vi "ReadNumeric.vi"(1 "reference":refnum<vi>) -> (0 "Numeric":T10)   [LabVIEW 2013]
uses:
  <vilib>/Utility/miscctls.llb/LVBoundsTypeDef.ctl
  <vilib>/Utility/miscctls.llb/LVRectTypeDef.ctl
  <vilib>/Utility/miscctls.llb/LVPositionTypeDef.ctl
  <vilib>/Utility/miscctls.llb/LVDataSocketStatusTypeDef.ctl
  <vilib>/Utility/miscctls.llb/LVKeyNavTypeDef.ctl
  <vilib>/Utility/miscctls.llb/LVMinMaxIncTypeDef.ctl
  <vilib>/Utility/miscctls.llb/LVKeyTypeDef.ctl
  <vilib>/numeric/LVNumericRepresentation.ctl
  <vilib>/Utility/miscctls.llb/LVOutOfRangeActionTypeDef.ctl
panel:
  out "error out":errorcluster
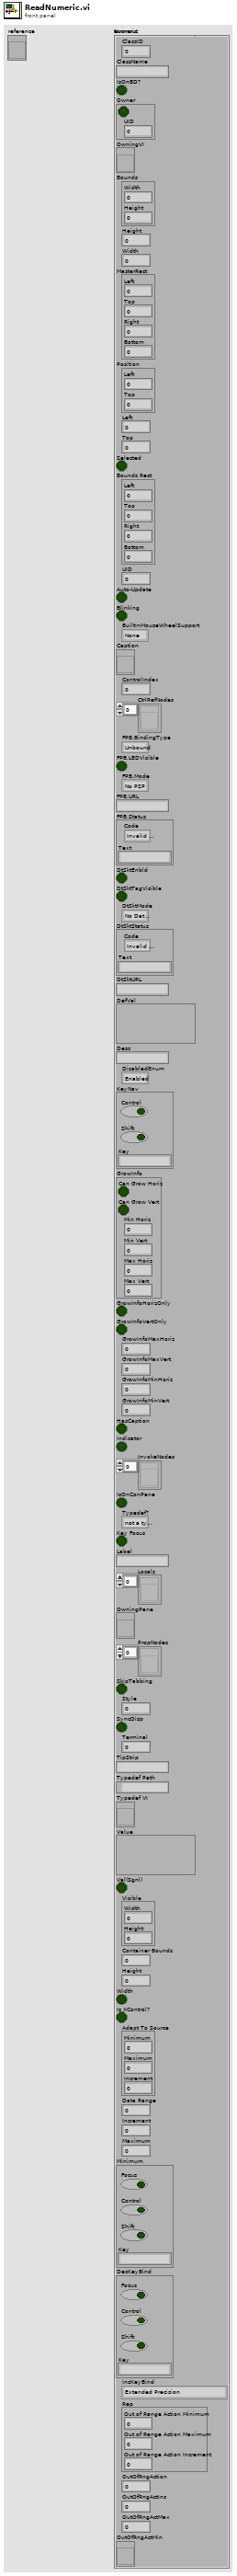
[diagram p1: front panel]
types:
  T1 = typedef "LVBoundsTypeDef.ctl" = cluster{"Width":u32, "Height":u32}
  T2 = typedef "LVRectTypeDef.ctl" = cluster{"Left":i16, "Top":i16, "Right":i16, "Bottom":i16}
  T3 = typedef "LVPositionTypeDef.ctl" = cluster{"Left":i32, "Top":i32}
  T4 = typedef "LVDataSocketStatusTypeDef.ctl" = cluster{"Code":enum32{"Invalid Status", "Unconnected", "Active", "Idle", "Error", "Connecting"}, "Text":string}
  T5 = typedef "LVKeyNavTypeDef.ctl" = cluster{"Control":bool, "Shift":bool, "Key":string}
  T6 = typedef "LVMinMaxIncTypeDef.ctl" = cluster{"Minimum":dbl, "Maximum":dbl, "Increment":dbl}
  T7 = typedef "LVKeyTypeDef.ctl" = cluster{"Focus":bool, "Control":bool, "Shift":bool, "Key":string}
  T8 = typedef "LVNumericRepresentation.ctl" = enum32{"Extended Precision", "Double Precision", "Single Precision", "Long", "Word", "Byte", "Unsigned Long", "Unsigned Word", "Unsigned Byte", "Complex Extended", "Complex Double", "Complex Single", "Quad", "Unsigned Quad", "Fixed-Point"}
  T9 = typedef "LVOutOfRangeActionTypeDef.ctl" = cluster{"Out of Range Action Minimum":u8, "Out of Range Action Maximum":u8, "Out of Range Action Increment":u8}
  T10 = cluster{"ClassID":u32, "ClassName":string, "IsOnBD?":bool, "Owner":cluster{bool, "UID":i32}, "OwningVI":refnum<vi>, "Bounds":T1, "Height":u32, "Width":u32, "MasterRect":T2, "Position":T3, "Left":i32, "Top":i32, "Selected":bool, "Bounds Rect":T2, "UID":i32, "Auto-Update":bool, "Blinking":bool, "BuiltInMouseWheelSupport":enum16{"None", "On Hover", "On Key Focus", "On Hover or Key Focus"}, "Caption":refnum<vi>, "ControlIndex":i32, "CtrlRefNodes":refnum<vi>[], "FPB.BindingType":enum32{"Unbound", "Bound To PSP URL", "Bound To Variable Shortcut"}, "FPB.LEDVisible":bool, "FPB.Mode":enum32{"No PSP", "Read", "Write", "Write & Read"}, "FPB.URL":string, "FPB.Status":T4, "DtSktEnbld":bool, "DtSktTagVisible":bool, "DtSktMode":enum32{"No DataSocket", "Publish", "Subscribe", "Publish & Subscribe"}, "DtSktStatus":T4, "DtSktURL":string, "DefVal":variant, "Desc":string, "DisabledEnum":enum8{"Enabled", "Disabled", "Disabled and Grayed Out"}, "KeyNav":T5, "GrowInfo":cluster{"Can Grow Horiz":bool, "Can Grow Vert":bool, "Min Horiz":i16, "Min Vert":i16, "Max Horiz":i16, "Max Vert":i16}, "GrowInfoHorizOnly":bool, "GrowInfoVertOnly":bool, "GrowInfoMaxHoriz":i16, "GrowInfoMaxVert":i16, "GrowInfoMinHoriz":i16, "GrowInfoMinVert":i16, "HasCaption":bool, "Indicator":bool, "InvokeNodes":refnum<vi>[], "IsOnConPane":bool, "Typedef?":enum32{"not a typedef", "typedef", "strict typedef", "class private data"}, "Key Focus":bool, "Label":string, "Locals":refnum<vi>[], "OwningPane":refnum<vi>, "PropNodes":refnum<vi>[], "SkipTabbing":bool, "Style":u32, "SyncDisp":bool, "Terminal":i32, "TipStrip":string, "Typedef Path":path, "Typedef VI":refnum<vi>, "Value":variant, "Val(Sgnl)":bool, "Visible":T1, "Container Bounds":u32, "Height":u32, "Width":bool, "Is XControl?":bool, "Adapt To Source":T6, "Data Range":dbl, "Increment":dbl, "Maximum":dbl, "Minimum":T7, "DecKeyBind":T7, "IncKeyBind":T8, "Rep":T9, "OutOfRngAction":u8, "OutOfRngActInc":u8, "OutOfRngActMax":u8, "OutOfRngActMin":refnum<vi>}
  T11 = enum16{"None", "On Hover", "On Key Focus", "On Hover or Key Focus"}
  T12 = enum32{"Unbound", "Bound To PSP URL", "Bound To Variable Shortcut"}
  T13 = enum32{"No PSP", "Read", "Write", "Write & Read"}
  T14 = enum32{"No DataSocket", "Publish", "Subscribe", "Publish & Subscribe"}
  T15 = enum8{"Enabled", "Disabled", "Disabled and Grayed Out"}
  T16 = cluster{"Can Grow Horiz":bool, "Can Grow Vert":bool, "Min Horiz":i16, "Min Vert":i16, "Max Horiz":i16, "Max Vert":i16}
  T17 = enum32{"not a typedef", "typedef", "strict typedef", "class private data"}
  T18 = cluster{"ClassID":u32, "ClassName":string, "IsOnBD?":bool, "Cluster":cluster{bool, "UID":i32}, "OwningVI":refnum<vi>, "Bounds":T1, "Height":u32, "Width":u32, "MasterRect":T2, "Position":T3, "Left":i32, "Top":i32, "Selected":bool, "Bounds Rect":T2, "UID":i32, "Auto-Update":bool, "Blinking":bool, "BuiltInMouseWheelSupport":enum16{"None", "On Hover", "On Key Focus", "On Hover or Key Focus"}, "Caption":refnum<vi>, "ControlIndex":i32, "CtrlRefNodes":refnum<vi>[], "FPB.BindingType":enum32{"Unbound", "Bound To PSP URL", "Bound To Variable Shortcut"}, "FPB.LEDVisible":bool, "FPB.Mode":enum32{"No PSP", "Read", "Write", "Write & Read"}, "FPB.URL":string, "FPB.Status":T4, "DtSktEnbld":bool, "DtSktTagVisible":bool, "DtSktMode":enum32{"No DataSocket", "Publish", "Subscribe", "Publish & Subscribe"}, "DtSktStatus":T4, "DtSktURL":string, "DefVal":variant, "Desc":string, "DisabledEnum":enum8{"Enabled", "Disabled", "Disabled and Grayed Out"}, "KeyNav":T5, "GrowInfo":cluster{"Can Grow Horiz":bool, "Can Grow Vert":bool, "Min Horiz":i16, "Min Vert":i16, "Max Horiz":i16, "Max Vert":i16}, "GrowInfoHorizOnly":bool, "GrowInfoVertOnly":bool, "GrowInfoMaxHoriz":i16, "GrowInfoMaxVert":i16, "GrowInfoMinHoriz":i16, "GrowInfoMinVert":i16, "HasCaption":bool, "Indicator":bool, "InvokeNodes":refnum<vi>[], "IsOnConPane":bool, "Typedef?":enum32{"not a typedef", "typedef", "strict typedef", "class private data"}, "Key Focus":bool, "Text":string, "Locals":refnum<vi>[], "OwningPane":refnum<vi>, "PropNodes":refnum<vi>[], "SkipTabbing":bool, "Style":u32, "SyncDisp":bool, "UID":i32, "TipStrip":string, "Typedef Path":path, "Typedef VI":refnum<vi>, "Value":variant, "Visible":bool, "Container Bounds":T1, "Height":u32, "Width":u32, "Is XControl?":bool, "Adapt To Source":bool, "Data Range":T6, "Increment":dbl, "Maximum":dbl, "Minimum":dbl, "DecKeyBind":T7, "IncKeyBind":T7, "Rep":T8, "OutOfRngAction":T9, "OutOfRngActInc":u8, "OutOfRngActMax":u8, "OutOfRngActMin":u8, "UnitLabel":refnum<vi>}
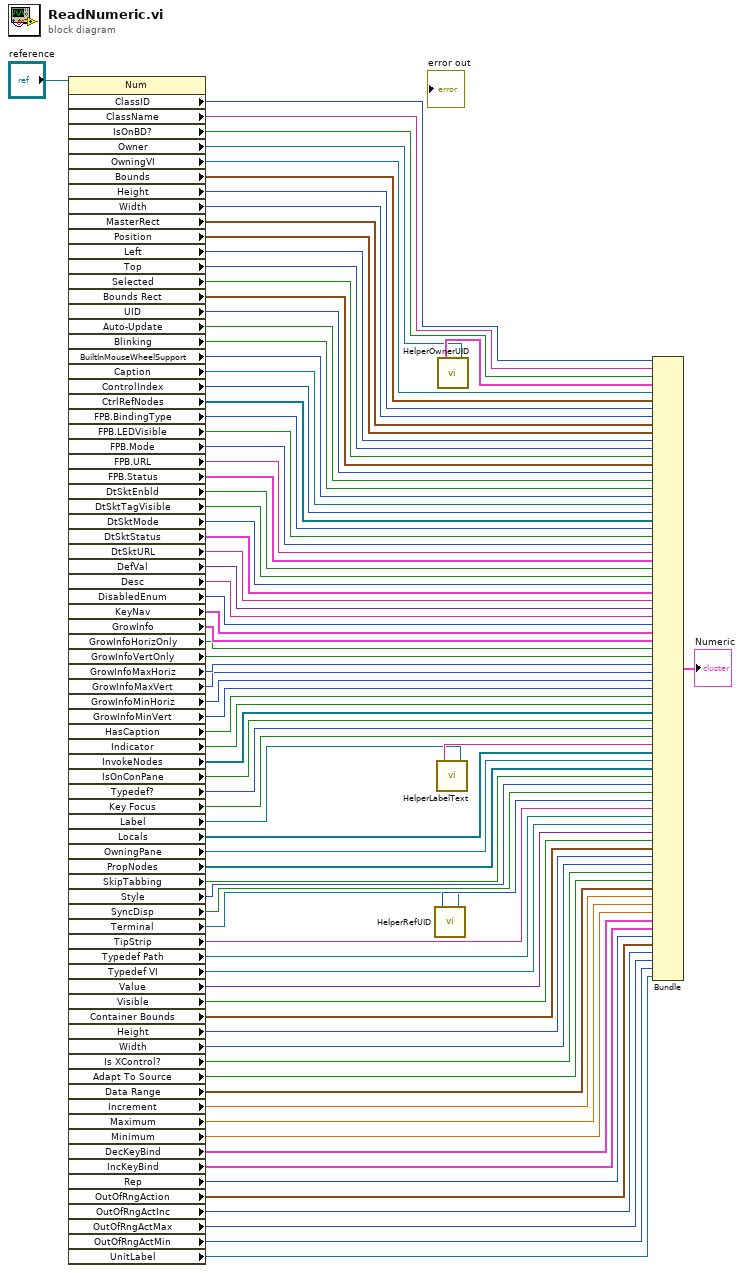
[diagram p0: block diagram]
diagram:
  n1 = property class="Num"(reference="reference") -> ("ClassID"=w82:u32, "ClassName"=w81:string, "IsOnBD?"=w80:bool, "Owner"=w78:refnum<vi>, "OwningVI"=w77:refnum<vi>, "Bounds"=w76:T1, "Height"=w75:u32, "Width"=w74:u32, "MasterRect"=w73:T2, "Position"=w72:T3, "Left"=w71:i32, "Top"=w70:i32, "Selected"=w69:bool, "Bounds Rect"=w68:T2, "UID"=w67:i32, "Auto-Update"=w66:bool, "Blinking"=w65:bool, "BuiltInMouseWheelSupport"=w64:T11, "Caption"=w63:refnum<vi>, "ControlIndex"=w62:i32, "CtrlRefNodes"=w61:refnum<vi>[], "FPB.BindingType"=w60:T12, "FPB.LEDVisible"=w59:bool, "FPB.Mode"=w58:T13, "FPB.URL"=w57:string, "FPB.Status"=w56:T4, "DtSktEnbld"=w55:bool, "DtSktTagVisible"=w54:bool, "DtSktMode"=w53:T14, "DtSktStatus"=w52:T4, "DtSktURL"=w51:string, "DefVal"=w50:variant, "Desc"=w49:string, "DisabledEnum"=w48:T15, "KeyNav"=w47:T5, "GrowInfo"=w46:T16, "GrowInfoHorizOnly"=w45:bool, "GrowInfoVertOnly"=w44:bool, "GrowInfoMaxHoriz"=w43:i16, "GrowInfoMaxVert"=w42:i16, "GrowInfoMinHoriz"=w41:i16, "GrowInfoMinVert"=w40:i16, "HasCaption"=w39:bool, "Indicator"=w38:bool, "InvokeNodes"=w37:refnum<vi>[], "IsOnConPane"=w36:bool, "Typedef?"=w35:T17, "Key Focus"=w34:bool, "Label"=w32:refnum<vi>, "Locals"=w31:refnum<vi>[], "OwningPane"=w30:refnum<vi>, "PropNodes"=w29:refnum<vi>[], "SkipTabbing"=w28:bool, "Style"=w27:u32, "SyncDisp"=w26:bool, "Terminal"=w24:refnum<vi>, "TipStrip"=w23:string, "Typedef Path"=w22:path, "Typedef VI"=w21:refnum<vi>, "Value"=w20:variant, "Visible"=w19:bool, "Container Bounds"=w18:T1, "Height"=w17:u32, "Width"=w16:u32, "Is XControl?"=w15:bool, "Adapt To Source"=w14:bool, "Data Range"=w13:T6, "Increment"=w12:dbl, "Maximum"=w11:dbl, "Minimum"=w10:dbl, "DecKeyBind"=w9:T7, "IncKeyBind"=w8:T7, "Rep"=w7:T8, "OutOfRngAction"=w6:T9, "OutOfRngActInc"=w5:u8, "OutOfRngActMax"=w4:u8, "OutOfRngActMin"=w3:u8, "UnitLabel"=w2:refnum<vi>)  [unwired: 1 in, 2 out]
  n2 = call "HelperRefUID.vi"("Text in"=w24) -> ("UID"=w25:i32)
  n3 = call "HelperLabelText.vi"("Text in"=w32) -> ("Text"=w33:string)
  n4 = call "HelperOwnerUID.vi"("Generic in"=w78) -> ("Cluster"=w79:cluster{bool, "UID":i32})
  n5 = Bundle("ClassID"=w82, "ClassName"=w81, "IsOnBD?"=w80, "Cluster"=w79, "OwningVI"=w77, "Bounds"=w76, "Height"=w75, "Width"=w74, "MasterRect"=w73, "Position"=w72, "Left"=w71, "Top"=w70, "Selected"=w69, "Bounds Rect"=w68, "UID"=w67, "Auto-Update"=w66, "Blinking"=w65, "BuiltInMouseWheelSupport"=w64, "Caption"=w63, "ControlIndex"=w62, "CtrlRefNodes"=w61, "FPB.BindingType"=w60, "FPB.LEDVisible"=w59, "FPB.Mode"=w58, "FPB.URL"=w57, "FPB.Status"=w56, "DtSktEnbld"=w55, "DtSktTagVisible"=w54, "DtSktMode"=w53, "DtSktStatus"=w52, "DtSktURL"=w51, "DefVal"=w50, "Desc"=w49, "DisabledEnum"=w48, "KeyNav"=w47, "GrowInfo"=w46, "GrowInfoHorizOnly"=w45, "GrowInfoVertOnly"=w44, "GrowInfoMaxHoriz"=w43, "GrowInfoMaxVert"=w42, "GrowInfoMinHoriz"=w41, "GrowInfoMinVert"=w40, "HasCaption"=w39, "Indicator"=w38, "InvokeNodes"=w37, "IsOnConPane"=w36, "Typedef?"=w35, "Key Focus"=w34, "Text"=w33, "Locals"=w31, "OwningPane"=w30, "PropNodes"=w29, "SkipTabbing"=w28, "Style"=w27, "SyncDisp"=w26, "UID"=w25, "TipStrip"=w23, "Typedef Path"=w22, "Typedef VI"=w21, "Value"=w20, "Visible"=w19, "Container Bounds"=w18, "Height"=w17, "Width"=w16, "Is XControl?"=w15, "Adapt To Source"=w14, "Data Range"=w13, "Increment"=w12, "Maximum"=w11, "Minimum"=w10, "DecKeyBind"=w9, "IncKeyBind"=w8, "Rep"=w7, "OutOfRngAction"=w6, "OutOfRngActInc"=w5, "OutOfRngActMax"=w4, "OutOfRngActMin"=w3, "UnitLabel"=w2) -> (→"Numeric":T18)  [unwired: 1 in]
